vi "运控模式.vi"() -> ()   [LabVIEW 2023]
uses:
  <vilib>/Instr/_visa.llb/VISA Configure Serial Port (Instr).vi
panel:
  out "读取缓冲区 2":string
  out "读取缓冲区":string
  in  "清空缓冲区":bool
  in  "电机ID":string
  out "错误输出":errorcluster
  in  "停止":bool
  in  "运控模式开始":bool
  in  "断开电机":bool
  in  "Kd":dbl(slide) scale=0.0..5.0 scale format="%#_4g"
  in  "Kp":dbl(slide) scale=0.0..500.0
  in  "速度":dbl(slide) scale=-30.0..30.0
  in  "扭矩":dbl(slide) scale=-12.0..12.0
  in  "位置":dbl(slide) scale=-12.5..12.5
  in  "baud rate (9600)":u32=921600 caption="波特率(9600)"
  in  "VISA resource name":refnum<visa-resource-name> caption="VISA资源名称"
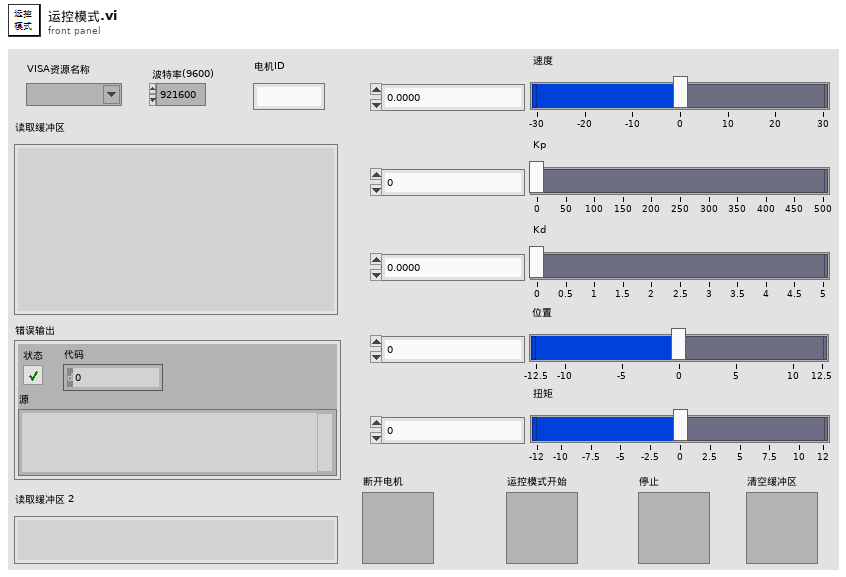
[diagram p1: front panel]
types:
  T1 = typedef "状态机.ctl" = enum16{"连接电机", "电机使能", "等待输入", "运控模式", "信息发送", "清空缓冲区", "停止", "断开"}
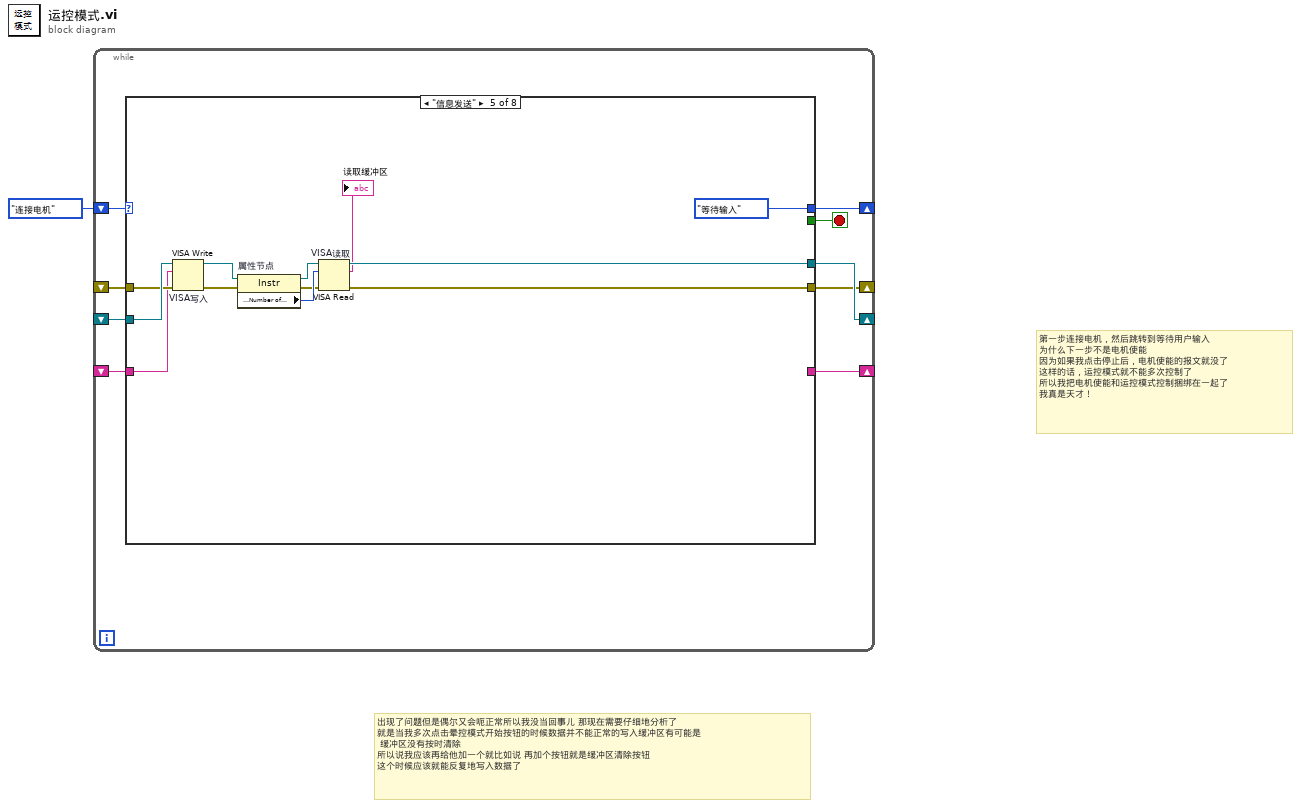
[diagram p0: block diagram]
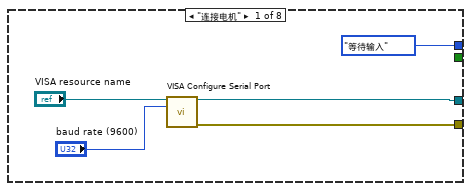
[diagram p2: hidden frame]
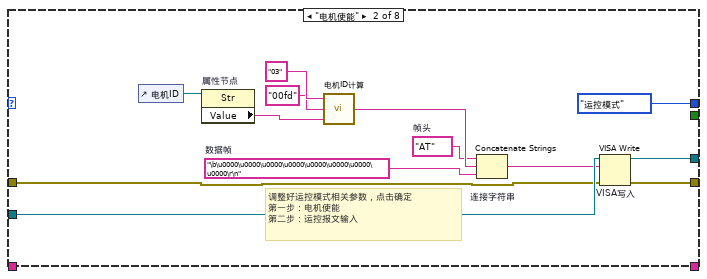
[diagram p3: hidden frame]
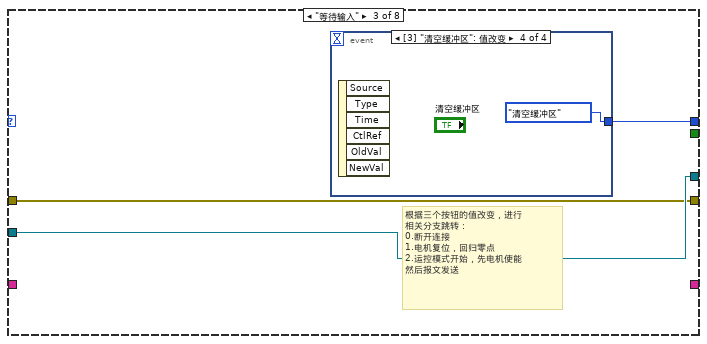
[diagram p4: hidden frame]
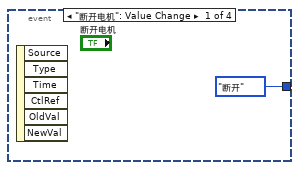
[diagram p5: hidden frame]
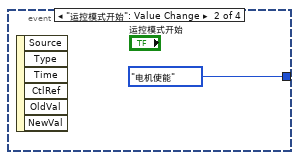
[diagram p6: hidden frame]
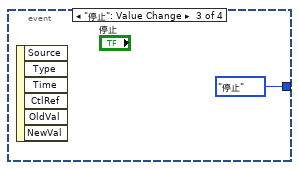
[diagram p7: hidden frame]
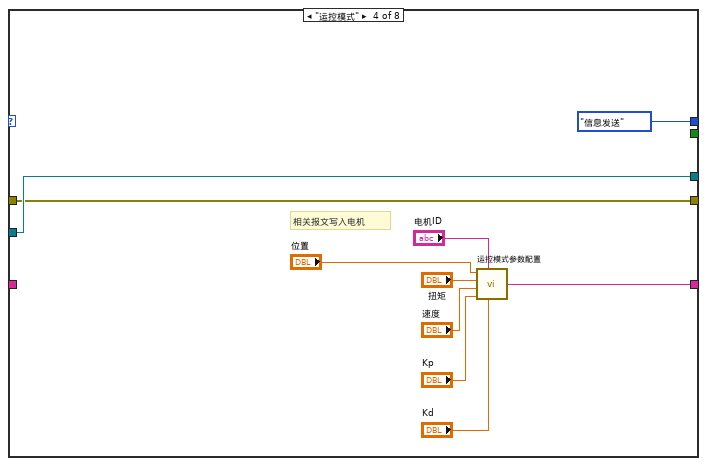
[diagram p8: hidden frame]
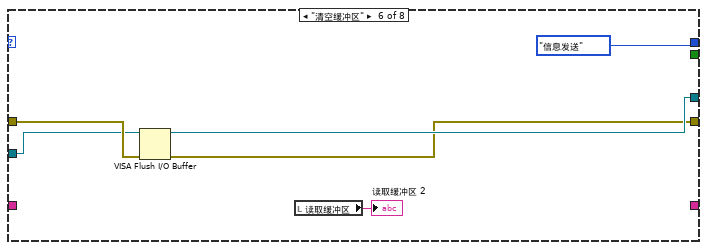
[diagram p9: hidden frame]
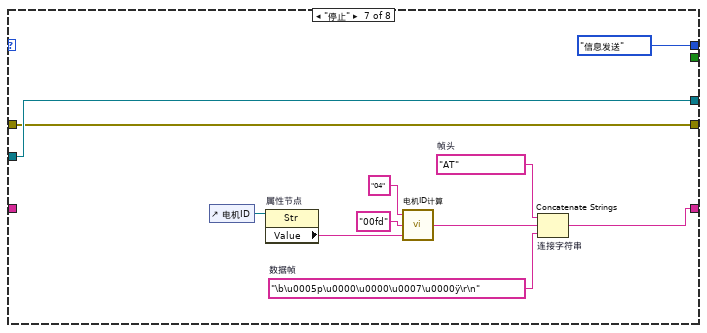
[diagram p10: hidden frame]
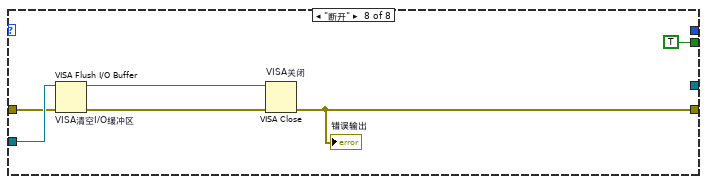
[diagram p11: hidden frame]
diagram:
  # "出现了问题但是偶尔又会呃正常所以我没当回事儿 那现在需要仔细地分析了 \n就是当我多次点击晕控模式开始按钮的时候数据并不能正常的写入缓冲区有可能是\n 缓冲区没有按时清除 \n所以说我应该再给他加一个就比如说 再加个按钮就是缓冲区清除按钮 \n这个时候应该就能反复地写入数据了"
  # "第一步连接电机，然后跳转到等待用户输入\n为什么下一步不是电机使能\n因为如果我点击停止后，电机使能的报文就没了\n这样的话，运控模式就不能多次控制了\n所以我把电机使能和运控模式控制捆绑在一起了\n我真是天才！"
  n1 = while {
    shift-right: [w10] -> _
    shift-left: _ -> [w9]
    shift-right: [w7] -> _
    shift-left: _ -> [w8]
    shift-right: [w3] -> _
    shift-left: 状态机."连接电机" -> [w5]
    shift-right: [w6] -> _
    shift-left: _ -> [w2]
    stop <- w4 stop-if-true
    n2 = case shown="\"信息发送\"" w5 {
      tunnel: [w13 w26 w30 w45 w53 w61 w73 _] -> w10
      tunnel: w9 -> [_ w28 w30 w45 w57 w62 w73 w79]
      tunnel: [_ _ _ w36 _ _ w66 _] -> w6
      tunnel: w8 -> [_ w27 w29 w44 w56 w63 w72 w78]
      tunnel: [w12 w25 w29 w44 w52 w60 w72 w76] -> w7
      tunnel: [_ _ _ _ _ _ _ TRUE] -> w4
      tunnel: [状态机."等待输入" 状态机."运控模式" w31 状态机."信息发送" 状态机."等待输入" 状态机."信息发送" 状态机."信息发送" _] -> w3
      tunnel: w2 -> [_ _ _ _ w55 _ _ _]
      frame "连接电机" {
        n3 = call-poly "VISA Configure Serial Port"("VISA resource name"="VISA resource name", "baud rate (9600)"="baud rate (9600)") -> ("VISA resource name out"=w13:refnum<visa-resource-name>, "error out"=w12:errorcluster)  [unwired: 12 in]
      }
      frame "电机使能" {
        w18 = "\b\u0000\u0000\u0000\u0000\u0000\u0000\u0000\u0000\r\n"  # 数据帧
        w17 = "AT"  # 帧头
        # "调整好运控模式相关参数，点击确定\n第一步：电机使能\n第二步：运控报文输入"
        n4 = control-ref of="电机ID"() -> (w21:refnum<vi>)
        n5 = property on="属性节点" class="Str"(reference=w21) -> ("Value"=w20:string)  [unwired: 1 in, 2 out]
        n6 = call "电机ID计算.vi"("电机ID"=w20, "主机id"="00fd", "通信模式"="03") -> ("最终输出报文"=w19:string)
        n7 = Concatenate Strings "连接字符串"(w17, w19, w18) -> (w16:string)
        n8 = VISA Write "VISA写入"(VISA resource name=w28, write buffer=w16, error in (no error)=w27) -> (VISA resource name out=w26:refnum<visa-resource-name>, error out=w25:errorcluster)  [unwired: 1 out]
      }
      frame "等待输入" {
        # "根据三个按钮的值改变，进行\n相关分支跳转：\n0.断开连接\n1.电机复位，回归零点\n2.运控模式开始，先电机使能\n然后报文发送"
        n9 = event shown="[3] \"清空缓冲区\": 值改变" {
          selector: _ -> [_ _ _ _]
          dyn-events: _ -> [_ _ _ _]
          timeout: _ -> [_ _ _ _]
          tunnel: [状态机."断开" 状态机."电机使能" 状态机."停止" 状态机."清空缓冲区"] -> w31
          event "断开电机": Value Change {
            n10 = event-data() -> ()  [unwired: 1 in, 6 out]
          }
          event "运控模式开始": Value Change {
            n11 = event-data() -> ()  [unwired: 1 in, 6 out]
          }
          event "停止": Value Change {
            n12 = event-data() -> ()  [unwired: 1 in, 6 out]
          }
          event "清空缓冲区": Value Change {
            n13 = event-data() -> ()  [unwired: 1 in, 6 out]
          }
        }
      }
      frame "运控模式" {
        # "相关报文写入电机"
        n14 = call "运控模式参数配置.vi"("Kd"="Kd", "电机ID"="电机ID", "Kp"="Kp", "速度"="速度", "扭矩"="扭矩", "位置"="位置") -> ("最终输出报文"=w36:string)
      }
      frame "信息发送" {
        n15 = VISA Write "VISA写入"(VISA resource name=w57, write buffer=w55, error in (no error)=w56) -> (VISA resource name out=w51:refnum<visa-resource-name>, error out=w48:errorcluster)  [unwired: 1 out]
        n16 = property on="属性节点" class="Instr"(reference=w51, error in=w48) -> (reference out=w50:refnum<visa-resource-name>, error out=w47:errorcluster, "Serial Settings:Number of Bytes at Serial Port"=w49:u32)
        n17 = VISA Read "VISA读取"(VISA resource name=w50, byte count=w49, error in (no error)=w47) -> (VISA resource name out=w53:refnum<visa-resource-name>, read buffer=→"读取缓冲区":string, error out=w52:errorcluster)  [unwired: 1 out]
      }
      frame "清空缓冲区" {
        n18 = VISA Flush I/O Buffer(VISA resource name=w62, error in (no error)=w63) -> (VISA resource name out=w61:refnum<visa-resource-name>, error out=w60:errorcluster)  [unwired: 1 in]
        n19 = local read "读取缓冲区"() -> (→"读取缓冲区 2":string)
      }
      frame "停止" {
        w67 = "\b\u0005p\u0000\u0000\u0007\u0000ÿ\r\n"  # 数据帧
        w69 = "AT"  # 帧头
        n20 = control-ref of="电机ID"() -> (w65:refnum<vi>)
        n21 = property on="属性节点" class="Str"(reference=w65) -> ("Value"=w64:string)  [unwired: 1 in, 2 out]
        n22 = call "电机ID计算.vi"("电机ID"=w64, "主机id"="00fd", "通信模式"="04") -> ("最终输出报文"=w68:string)
        n23 = Concatenate Strings "连接字符串"(w69, w68, w67) -> (w66:string)
      }
      frame "断开" {
        n24 = VISA Flush I/O Buffer "VISA清空I/O缓冲区"(VISA resource name=w79, error in (no error)=w78) -> (VISA resource name out=w77:refnum<visa-resource-name>, error out=w75:errorcluster)  [unwired: 1 in]
        n25 = VISA Close "VISA关闭"(VISA resource name=w77, error in (no error)=w75) -> (error out=w76:errorcluster)
        "错误输出" <- w76
      }
    }
  }
